vi "Scostamento%.vi"(10 "media":dbl, 11 "valore":dbl) -> (3 "Scostamento %":dbl)   [LabVIEW 2019]
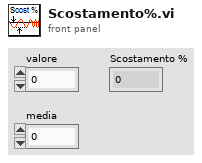
[diagram p1: front panel]
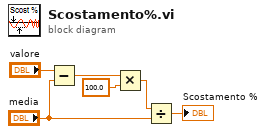
[diagram p0: block diagram]
diagram:
  n1 = Subtract(x="valore", y="media") -> (x-y=w4:dbl)
  n2 = Multiply(x=w4, y=100.0) -> (x*y=w2:dbl)
  n3 = Divide(x=w2, y="media") -> (x/y=→"Scostamento %":dbl)
